vi "exemploRW.vi"() -> ()   [LabVIEW 2019]
panel:
  out "Data 2":dbl
  in  "Função de Leitura":i32(ring)=2 items=["Zero in progress", "Perform flowmeter zeroing", "Mass flow rate", "Density", "Temperature", "Volume flow rate", "Pressure (internally derived)", "Mass total", "Volume total", "Mass inventory", "Volume inventory", "Start/stop all totalizers", "Reset all totalizers", "Reset all inventories", "Real-time interrupt failure", "Sensor failure", "Temperature sensor failure", "Flowmeter zeroing failure", "Other failure occurred", "Mass flow rate meter factor", "Volume flow rate meter factor", "Density meter factor", "Flowing density calibration constant", "Mass flow scale factor", "Density scale factor", "Temperature scale factor", "Volume flow scale factor", "Pressure scale factor", "Mass total scale factor", "Volume total scale factor", "Mass inventory scale factor", "Volume inventory scale factor", "Flowmeter zeroing standard deviantion (units in microsec)", "Standard or special mass flow unit", "Density unit", "Temperature unit", "Standard or special volume flow unit", "Pressure unit", "Standard or special mass total or inventory unit", "Standard or special volume total or inventory unit", "Base mass unit for special mass unit", "Base time uni for special mass unit", "Base volume unit for special volume unit", "Base time unit for special volume unit", "Maximum zeroing time", "Flow direction", "EEProm checksum failure", "EEProm checksum failure in core processor", "EEProm database corrupt", "RAM diagnostic failure", "RAM diagnostic failure in core processor", "Real-time Interrupt failure", "Watchdog timer error", "Mass flow cutoff", "Volume flow cutoff", "Integer de erro 001", "Slug flow high-density limit (g/cm3)", "Slug flow low-density limit (g/cm3)"]
  in  "Data":dbl
  in  "Função de Escrita":i32(ring) items=["Perform flowmeter zeroing", "Start/stop all totalizers", "Reset all totalizers", "Reset all inventories", "Mass flow rate meter factor", "Volume flow rate meter factor", "Density meter factor", "Flowing density calibration constant", "Mass flow scale factor", "Density scale factor", "Temperature scale factor", "Volume flow scale factor", "Pressure scale factor", "Mass total scale factor", "Volume total scale factor", "Mass inventory scale factor", "Volume inventory scale factor", "Standard or special mass flow unit", "Density unit", "Temperature unit", "Standard or special volume flow unit", "Pressure unit", "Standard or special mass total or inventory unit", "Standard or special volume total or inventory unit", "Base mass unit for special mass unit", "Base time uni for special mass unit", "Base volume unit for special volume unit", "Base time unit for special volume unit", "Maximum zeroing time", "Flow direction", "Perform transmitter self-test", "Mass flow cutoff", "Volume flow cutoff", "Slug flow high-density limit (g/cm3)", "Slug flow low-density limit (g/cm3)"]
  out "Waveform Chart":dbl(graph)
  in  "OK Button":bool
  in  "stop":bool
  out "Vazão Mássica [kg/h]":dbl
  out "Erro Fluximetro":errorcluster
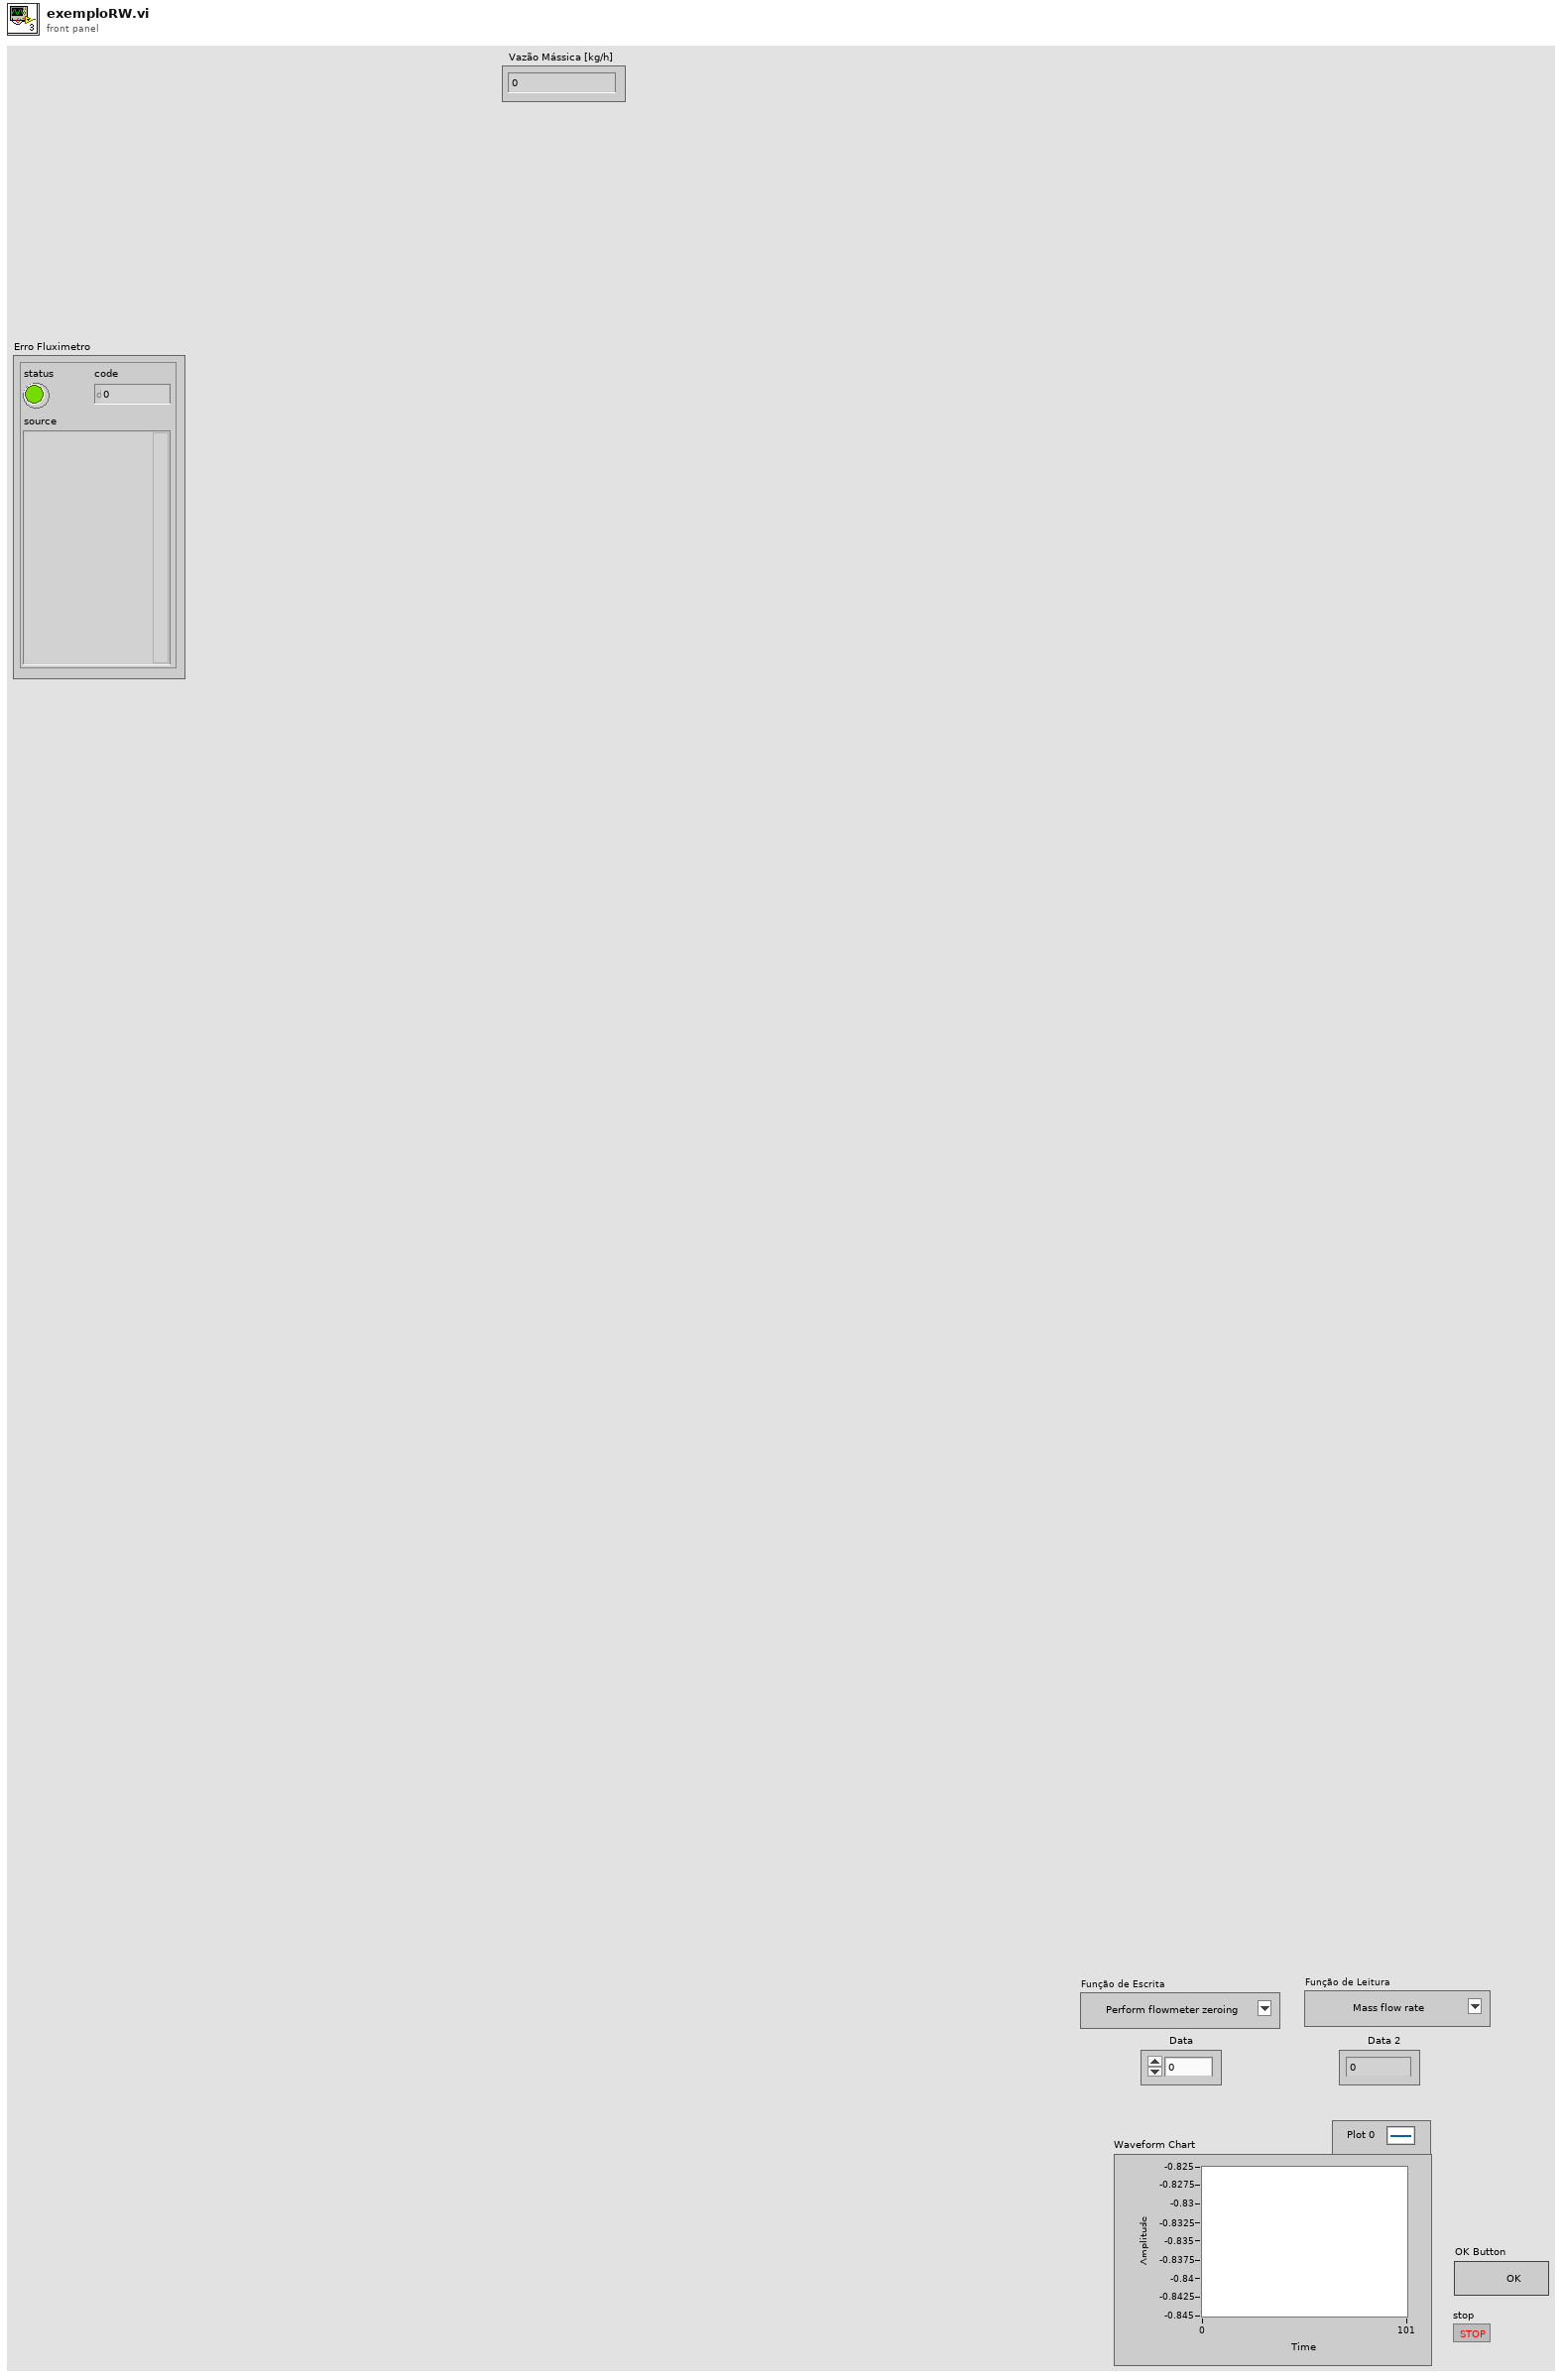
[diagram p1: front panel]
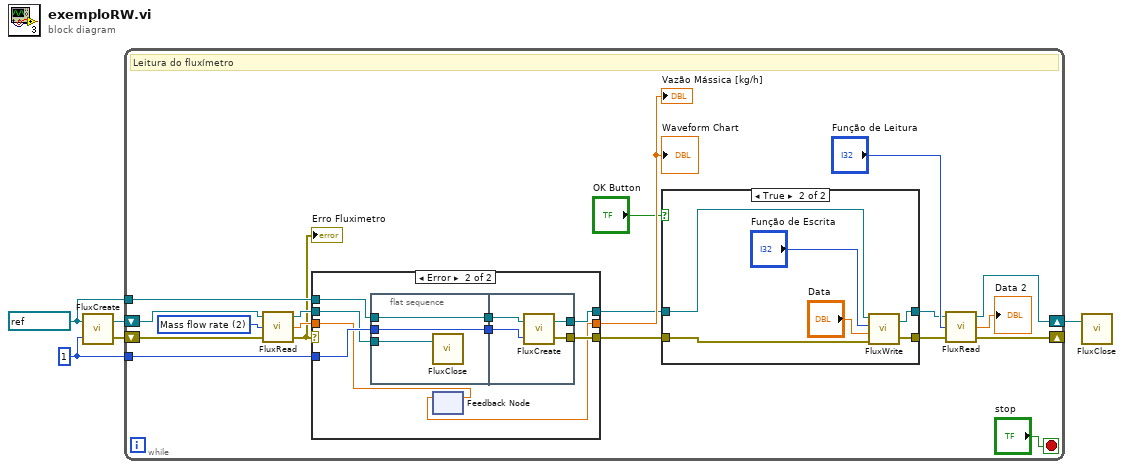
[diagram p0: block diagram]
diagram:
  w2 = refnum<visa-resource-name> "COM3" ("VISA resource")
  w1 = u16 1 ("Endereço slave")
  n1 = call "FluxCreate.vi"("Endereço slave"=w1, "Recurso VISA"=w2) -> ("Error Out"=w4:errorcluster, "Master Out"=w3:refnum<class "Modbus Master.lvclass">)
  n2 = while {
    shift-right: [w8] -> w5
    shift-left: w3 -> [w20]
    tunnel: w1 -> [w23]
    tunnel: w2 -> [w22]
    shift-right: [w9] -> _
    shift-left: w4 -> [w21]
    stop <- "stop" stop-if-true
    w24 = 2 items=["Zero in progress", "Perform flowmeter zeroing", "Mass flow rate", "Density", "Temperature", "Volume flow rate", "Pressure (internally derived)", "Mass total", "Volume total", "Mass inventory", "Volume inventory", "Start/stop all totalizers", "Reset all totalizers", "Reset all inventories", "Real-time interrupt failure", "Sensor failure", "Temperature sensor failure", "Flowmeter zeroing failure", "Other failure occurred", "Mass flow rate meter factor", "Volume flow rate meter factor", "Density meter factor", "Flowing density calibration constant", "Mass flow scale factor", "Density scale factor", "Temperature scale factor", "Volume flow scale factor", "Pressure scale factor", "Mass total scale factor", "Volume total scale factor", "Mass inventory scale factor", "Volume inventory scale factor", "Flowmeter zeroing standard deviantion (units in microsec)", "Standard or special mass flow unit", "Density unit", "Temperature unit", "Standard or special volume flow unit", "Pressure unit", "Standard or special mass total or inventory unit", "Standard or special volume total or inventory unit", "Base mass unit for special mass unit", "Base time uni for special mass unit", "Base volume unit for special volume unit", "Base time unit for special volume unit", "Maximum zeroing time", "Flow direction", "EEProm checksum failure", "EEProm checksum failure in core processor", "EEProm database corrupt", "RAM diagnostic failure", "RAM diagnostic failure in core processor", "Real-time Interrupt failure", "Watchdog timer error", "Mass flow cutoff", "Volume flow cutoff", "Integer de erro 001", "Slug flow high-density limit (g/cm3)", "Slug flow low-density limit (g/cm3)"] ("Descrição da função leitura")
    # "Leitura do fluxímetro"
    n3 = call "FluxRead.vi"("Error In"=w21, "Função de Leitura"=w24, "Master In"=w20) -> ("Error Out"=w17:errorcluster, "Data"=w18:dbl, "Master Out"=w19:refnum<class "Modbus Master.lvclass">)
    "Erro Fluximetro" <- w17
    n4 = case shown="Error" w17 {
      selector: w17 -> [w34 _]
      tunnel: w19 -> [w35 w38]
      tunnel: [w35 w44] -> w14
      tunnel: [w34 w41] -> w13
      tunnel: w23 -> [_ w43]
      tunnel: w22 -> [_ w42]
      tunnel: w18 -> [w33 w37]
      tunnel: [w33 w36] -> w15
      frame No Error {
      }
      frame Error {
        n5 = flat-sequence {
          tunnel: w42 -> [w46]
          tunnel: w43 -> [w47]
          tunnel: [w47] -> w40
          tunnel: [w46] -> w39
          tunnel: w38 -> [w45]
          tunnel: [w51] -> w44
          tunnel: [w48] -> w41
          tunnel: w40 -> [w50]
          tunnel: w39 -> [w49]
          frame #0 {
            n6 = call "FluxClose.vi"("Master In"=w45) -> ()  [unwired: 1 in, 1 out]
          }
          frame #1 {
            n7 = call "FluxCreate.vi"("Endereço slave"=w50, "Recurso VISA"=w49) -> ("Error Out"=w48:errorcluster, "Master Out"=w51:refnum<class "Modbus Master.lvclass">)
          }
        }
        n8 = feedback-in #1(w37) -> ()
        n9 = feedback #1() -> (w36:dbl)  [unwired: 1 in]
      }
    }
    "Vazão Mássica [kg/h]" <- w15
    "Waveform Chart" <- w15
    n10 = case shown="True" "OK Button" {
      tunnel: [w26 w28] -> w7
      tunnel: w14 -> [w26 w32]
      tunnel: w13 -> [w25 w31]
      tunnel: [w25 w27] -> w6
      frame False {
      }
      frame True {
        n11 = call "FluxWrite.vi"("Error In"=w31, "Data"="Data", "Função de Escrita"="Função de Escrita", "Master In"=w32) -> ("Error Out"=w27:errorcluster, "Master Out"=w28:refnum<class "Modbus Master.lvclass">)
      }
    }
    n12 = call "FluxRead.vi"("Error In"=w6, "Função de Leitura"="Função de Leitura", "Master In"=w7) -> ("Error Out"=w9:errorcluster, "Data"=→"Data 2":dbl, "Master Out"=w8:refnum<class "Modbus Master.lvclass">)
  }
  n13 = call "FluxClose.vi"("Master In"=w5) -> ()  [unwired: 1 in, 1 out]
